vi "RT Parse properties.vi"(8 "error in (no error)":errorcluster, 11 "Device Reference":T2 format="%.0x") -> (0 "error out":errorcluster, 1 "Write Block Descriptors":T1[](array[typedef]), 2 "Read Block Descriptors":T1[](array[typedef]), 3 "Device Ref out":T2 format="%.0x", 4 "Write":bool, 5 "max channel count bytes":u32, 6 "Read":bool)   [LabVIEW 2017, in "RefMem DMA Custom Device.lvlib"]
uses:
  RefMem DMA Custom Device.lvlib
  <vilib>/NI Veristand/Custom Device API/Custom Device Item Ref.ctl
  Block descriptor.ctl
  Controls/Data Channel Type.ctl
  <vilib>/NI Veristand/Custom Device API/Get Item Property (U32).vi
  <vilib>/NI Veristand/Custom Device Tools/Custom Device Utility Library/NI VeriStand - Search for All Items by Property.vi
  <vilib>/NI Veristand/Custom Device API/Get Item Property (U16).vi
  Controls/Global.vi
  <vilib>/NI Veristand/Custom Device Tools/Custom Device Utility Library/NI VeriStand - Search for All Items by GUID.vi
  <vilib>/NI VeriStand/Custom Device Tools/Custom Device Utility Library/Custom Device Utility Library.lvlib
  <vilib>/NI Veristand/Custom Device API/Custom Device API.lvlib
panel:
  out "error out 2":errorcluster
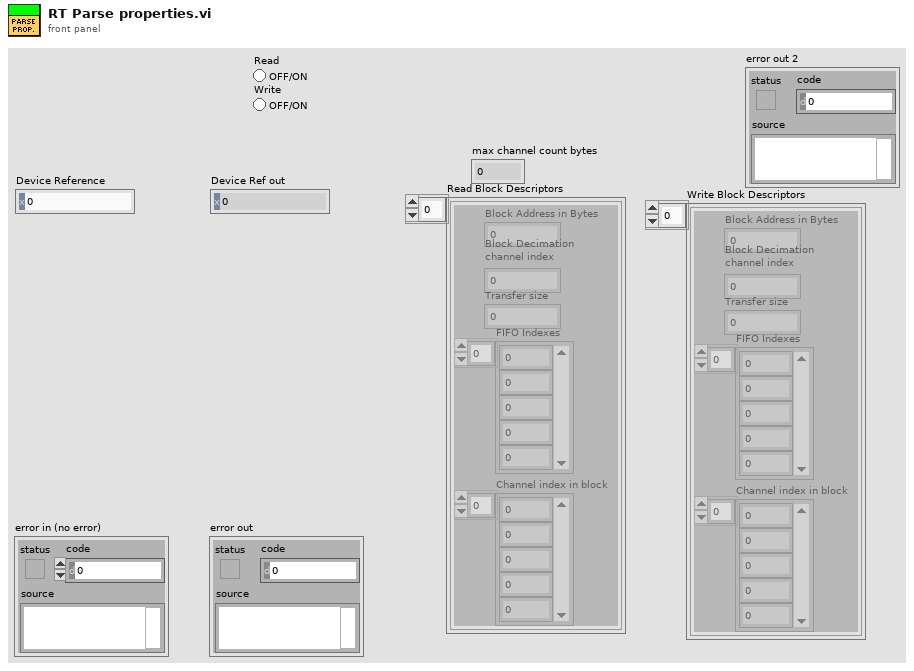
[diagram p1: front panel]
types:
  T1 = typedef "RefMem DMA Custom Device.lvlib/Block descriptor.ctl" = cluster{"Block Address in Bytes":u32, "Block Decimation \nchannel index":i32, "Transfer size":u32, "FIFO Indexes":i32[], "Channel index in block":i32[]}
  T2 = typedef "Custom Device API.lvlib/Custom Device Item Ref.ctl" = u64
  T3 = typedef "RefMem DMA Custom Device.lvlib/Data Channel Type.ctl" = enum16{"Read", "Write"}
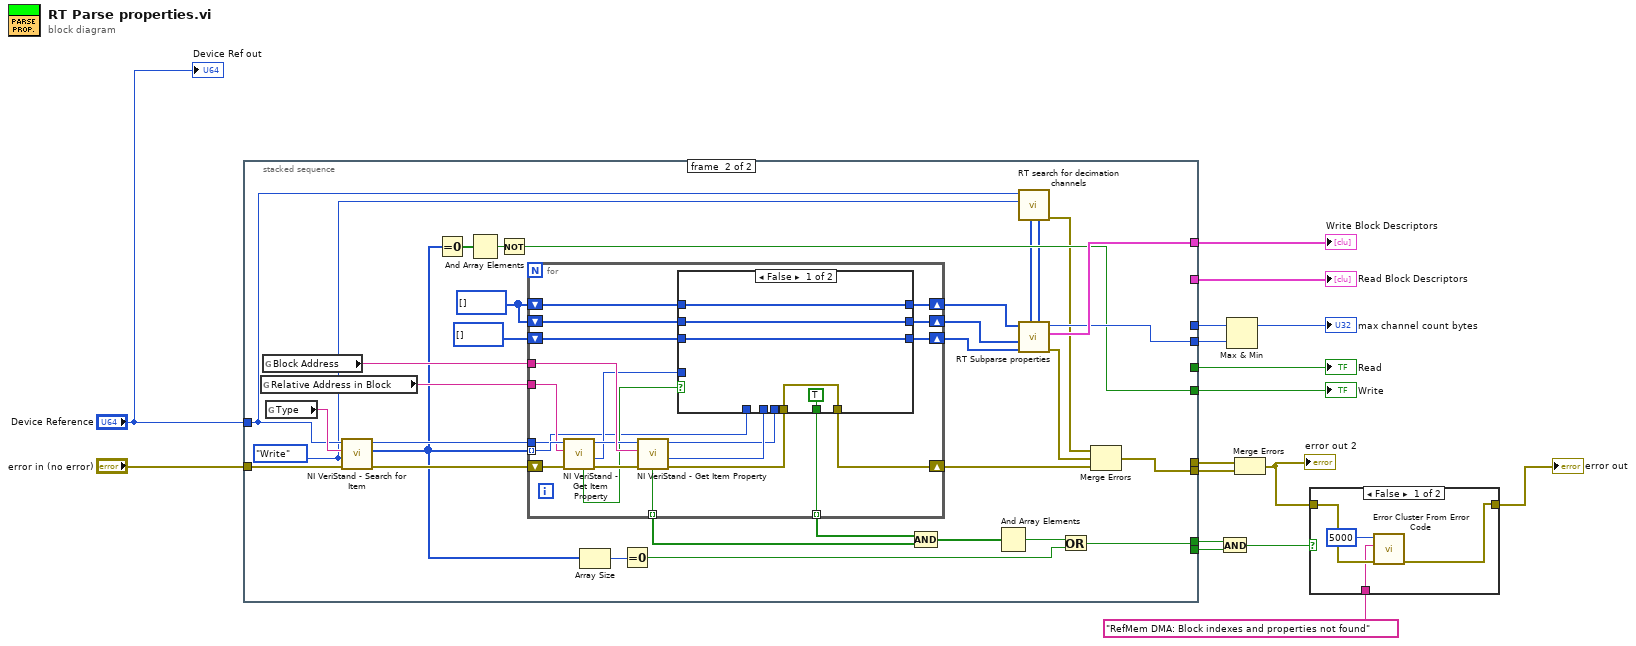
[diagram p0: block diagram]
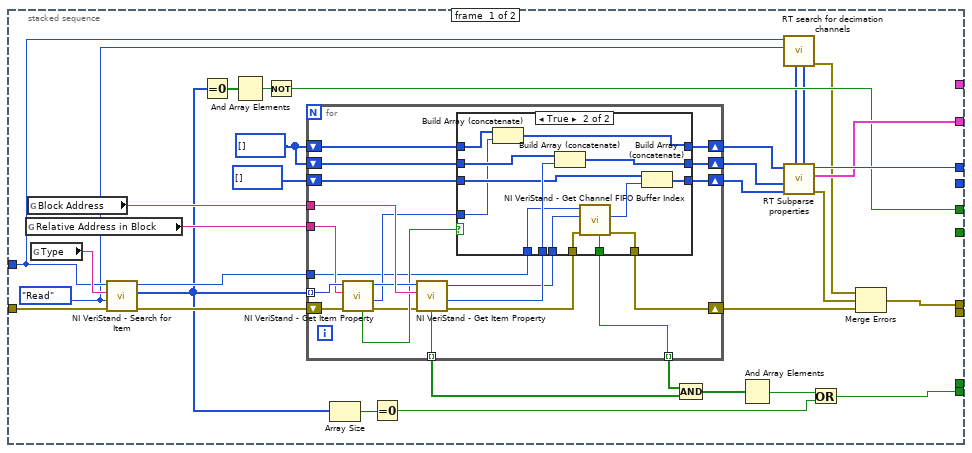
[diagram p2: hidden frame]
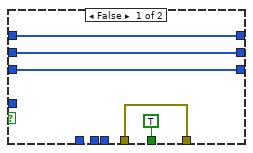
[diagram p3: hidden frame]
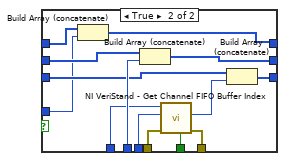
[diagram p4: hidden frame]
diagram:
  n1 = stacked-sequence {
    tunnel: "error in (no error)" -> [w49 w121]
    tunnel: [_ w90] -> w6
    tunnel: [w48 _] -> w9
    tunnel: "Device Reference" -> [w27 w99]
    tunnel: [w34 _] -> w12
    tunnel: [w46 _] -> w15
    tunnel: [w35 _] -> w14
    tunnel: [_ w113] -> w11
    tunnel: [_ w116] -> w10
    tunnel: [_ w115] -> w8
    tunnel: [w18 _] -> w4
    tunnel: [_ w114] -> w3
    frame #0 {
      w29 = u32[] []
      w26 = Data_Channel_Type."Read" ("DataChan Type")
      n2 = global read "Global.vi" "Relative Address in Block"() -> (w45:string)
      n3 = global read "Global.vi" "Block Address"() -> (w42:string)
      n4 = global read "Global.vi" "Type"() -> (w43:string)
      n5 = call-poly <vilib>:"NI VeriStand - Search for Item.vi"("error in"=w49, "Property Value"=w26, "Property Name"=w43, "Section Ref in"=w27) -> ("error out"=w41:errorcluster, "Item Refs"=w21:T2[], "Section Ref out"=w44:T2)  [unwired: 4 in, 1 out]
      n6 = Equal To 0?(x=w21) -> (x = 0?=w40:bool[])
      n7 = And Array Elements(Boolean array=w40) -> (logical AND=w47:bool)
      n8 = Not(x=w47) -> (.not. x?=w34:bool)
      n9 = for {
        tunnel: w21 -> [w69] mode=indexing
        tunnel: w45 -> [w68]
        shift-right: [w53] -> w36
        shift-left: w41 -> [w70]
        tunnel: w44 -> [w51]
        tunnel: [w52] -> w38 mode=indexing
        tunnel: w42 -> [w67]
        tunnel: [w66] -> w39 mode=indexing
        shift-right: [w61] -> w32
        shift-left: w29 -> [w64]
        shift-right: [w60] -> w31
        shift-left: w29 -> [w63]
        shift-right: [w59] -> w30
        shift-left: i32[] [] -> [w62]
        n10 = call-poly <vilib>:"NI VeriStand - Get Item Property.vi"("error in (no error)"=w70, "Property Name"=w68, "Item Ref in"=w69) -> ("error out"=w55:errorcluster, "Value"=w58:u32, "Item Ref out"=w65:T2, "Found?"=w56:bool)  [unwired: 5 in]
        n11 = call-poly <vilib>:"NI VeriStand - Get Item Property.vi"("error in (no error)"=w55, "Property Name"=w67, "Item Ref in"=w65) -> ("error out"=w54:errorcluster, "Value"=w57:u32, "Item Ref out"=w50:T2, "Found?"=w66:bool)  [unwired: 5 in]
        n12 = case shown="True" w56 {
          tunnel: [w75 w83] -> w61
          tunnel: w64 -> [w75 w89]
          tunnel: [w74 w86] -> w60
          tunnel: w63 -> [w74 w87]
          tunnel: [w73 w84] -> w59
          tunnel: w62 -> [w73 w85]
          tunnel: w57 -> [_ w88]
          tunnel: w58 -> [_ w82]
          tunnel: w54 -> [w71 w81]
          tunnel: [w71 w79] -> w53
          tunnel: [TRUE ("Found") w78] -> w52
          tunnel: w51 -> [_ w77]
          tunnel: w50 -> [_ w76]
          frame False {
          }
          frame True {
            n13 = Build Array (concatenate)(w89, w82) -> (w83:u32[])
            n14 = Build Array (concatenate)(w87, w88) -> (w86:u32[])
            n15 = call <vilib>:"NI VeriStand - Get Channel FIFO Buffer Index.vi"("error in"=w81, "Channel Ref"=w76, "Device Ref in"=w77) -> ("error out"=w79:errorcluster, "Channel FIFO Buffer Index"=w80:i32, "Found"=w78:bool)  [unwired: 4 in, 2 out]
            n16 = Build Array (concatenate)(w85, w80) -> (w84:i32[])
          }
        }
      }
      n17 = Array Size(array=w21) -> (size(s)=w20:i32)
      n18 = Equal To 0?(x=w20) -> (x = 0?=w19:bool)
      n19 = Compound Arithmetic op=AND(w38, w39) -> (w33:bool[])
      n20 = And Array Elements(Boolean array=w33) -> (logical AND=w22:bool)
      n21 = call "RT search for decimation channels.vi"("DataChan Type"=w26, "Device Reference"=w27) -> ("error out"=w25:errorcluster, "FIFO Index Decimation Table"=w23:i32[], "Block Address decimation table"=w24:u32[])  [unwired: 7 in]
      n22 = call "RT Subparse properties.vi"("FIFO Index Decimation Table"=w23, "Block Address decimation table"=w24, "FIFO indexes"=w30, "Block Address"=w31, "Relative Address in Block"=w32) -> ("error out"=w37:errorcluster, "Array out"=w46:T1[], "max block size"=w48:u32)  [unwired: 4 in]
      n23 = Or(x=w22, y=w19) -> (x .or. y?=w18:bool)
      n24 = Merge Errors(w25, w37, w36) -> (w35:errorcluster)
    }
    frame #1 {
      w102 = u32[] []
      w98 = Data_Channel_Type."Write" ("DataChan Type")
      n25 = global read "Global.vi" "Relative Address in Block"() -> (w110:string)
      n26 = global read "Global.vi" "Block Address"() -> (w111:string)
      n27 = global read "Global.vi" "Type"() -> (w120:string)
      n28 = call-poly <vilib>:"NI VeriStand - Search for Item.vi"("error in"=w121, "Property Value"=w98, "Property Name"=w120, "Section Ref in"=w99) -> ("error out"=w109:errorcluster, "Item Refs"=w91:T2[], "Section Ref out"=w108:T2)  [unwired: 4 in, 1 out]
      n29 = Equal To 0?(x=w91) -> (x = 0?=w119:bool[])
      n30 = And Array Elements(Boolean array=w119) -> (logical AND=w117:bool)
      n31 = Not(x=w117) -> (.not. x?=w113:bool)
      n32 = for {
        tunnel: w91 -> [w141] mode=indexing
        tunnel: w110 -> [w140]
        shift-right: [w125] -> w104
        shift-left: w109 -> [w142]
        tunnel: w108 -> [w124]
        tunnel: w111 -> [w139]
        tunnel: [w138] -> w103 mode=indexing
        shift-right: [w132] -> w107
        shift-left: w102 -> [w135]
        shift-right: [w131] -> w106
        shift-left: w102 -> [w134]
        shift-right: [w130] -> w105
        shift-left: i32[] [] -> [w133]
        tunnel: [w122] -> w100 mode=indexing
        n33 = call-poly <vilib>:"NI VeriStand - Get Item Property.vi"("error in (no error)"=w142, "Property Name"=w140, "Item Ref in"=w141) -> ("error out"=w136:errorcluster, "Value"=w129:u32, "Item Ref out"=w137:T2, "Found?"=w127:bool)  [unwired: 5 in]
        n34 = call-poly <vilib>:"NI VeriStand - Get Item Property.vi"("error in (no error)"=w136, "Property Name"=w139, "Item Ref in"=w137) -> ("error out"=w126:errorcluster, "Value"=w128:u32, "Item Ref out"=w123:T2, "Found?"=w138:bool)  [unwired: 5 in]
        n35 = case shown="False" w127 {
          tunnel: [w147 w155] -> w132
          tunnel: w135 -> [w147 w161]
          tunnel: [w146 w158] -> w131
          tunnel: w134 -> [w146 w159]
          tunnel: [w145 w156] -> w130
          tunnel: w133 -> [w145 w157]
          tunnel: w128 -> [_ w160]
          tunnel: w129 -> [_ w154]
          tunnel: w126 -> [w144 w153]
          tunnel: [w144 w152] -> w125
          tunnel: w124 -> [_ w151]
          tunnel: w123 -> [_ w150]
          tunnel: [TRUE ("Found") w148] -> w122
          frame False {
          }
          frame True {
            n36 = Build Array (concatenate)(w161, w154) -> (w155:u32[])
            n37 = Build Array (concatenate)(w159, w160) -> (w158:u32[])
            n38 = call <vilib>:"NI VeriStand - Get Channel FIFO Buffer Index.vi"("error in"=w153, "Channel Ref"=w150, "Device Ref in"=w151) -> ("error out"=w152:errorcluster, "Channel FIFO Buffer Index"=w149:i32, "Found"=w148:bool)  [unwired: 4 in, 2 out]
            n39 = Build Array (concatenate)(w157, w149) -> (w156:i32[])
          }
        }
      }
      n40 = Array Size(array=w91) -> (size(s)=w94:i32)
      n41 = Equal To 0?(x=w94) -> (x = 0?=w92:bool)
      n42 = Compound Arithmetic op=AND(w100, w103) -> (w112:bool[])
      n43 = And Array Elements(Boolean array=w112) -> (logical AND=w93:bool)
      n44 = call "RT search for decimation channels.vi"("DataChan Type"=w98, "Device Reference"=w99) -> ("error out"=w95:errorcluster, "FIFO Index Decimation Table"=w96:i32[], "Block Address decimation table"=w97:u32[])  [unwired: 7 in]
      n45 = call "RT Subparse properties.vi"("FIFO Index Decimation Table"=w96, "Block Address decimation table"=w97, "FIFO indexes"=w105, "Block Address"=w106, "Relative Address in Block"=w107) -> ("error out"=w118:errorcluster, "Array out"=w116:T1[], "max block size"=w115:u32)  [unwired: 4 in]
      n46 = Or(x=w93, y=w92) -> (x .or. y?=w90:bool)
      n47 = Merge Errors(w95, w118, w104) -> (w114:errorcluster)
    }
  }
  "Read Block Descriptors" <- w15
  "Read" <- w12
  "Write" <- w11
  "Write Block Descriptors" <- w10
  n48 = And(x=w6, y=w4) -> (x .and. y?=w5:bool)
  n49 = Max & Min(x=w9, y=w8) -> (max(x,y)=→"max channel count bytes":u32)  [unwired: 1 out]
  n50 = Merge Errors(w14, w3) -> (w13:errorcluster)
  "error out 2" <- w13
  n51 = case shown="False" w5 {
    tunnel: [w164 w166] -> w17
    tunnel: w13 -> [w165 w166]
    tunnel: "RefMem DMA: Block indexes and properties not found" ("error message (\"\")") -> [w162 _]
    frame False {
      n52 = call <vilib>:"Error Cluster From Error Code.vi"("error in (no error)"=w165, "error message (\"\")"=w162, "error code (0)"=5000) -> ("error out"=w164:errorcluster)  [unwired: 6 in]
    }
    frame True {
    }
  }
  "error out" <- w17
  "Device Ref out" <- "Device Reference"
